vi "TEST_LvMarkdown.vi"() -> ()   [LabVIEW 2021, in "LvMarkdown.lvlib"]
uses:
  LvMarkdown.lvlib
  TEST_LvMarkdownStep.ctl
  LvMarkdown/LineBreak/LineBreak.lvclass
  C:/GitHub/LvMarkdown/src/LvMarkdown/IRenderable/IRenderable.lvclass
  LvMarkdown/Collection/Collection.lvclass
  LvMarkdown/Heading/Heading.lvclass
  C:/GitHub/LvMarkdown/src/LvMarkdown/Markdown.lvclass
  LvMarkdown/Heading/Heading.lvclass/Heading.ctl
  LvMarkdown/Paragraph/Paragraph.lvclass
  LvMarkdown/Line/Line.lvclass
  LvMarkdown/HorizontalRule/HorizontalRule.lvclass
  LvMarkdown/Code/Code.lvclass
  LvMarkdown/Bold/Bold.lvclass
  LvMarkdown/Italic/Italic.lvclass
  LvMarkdown/Blockquote/Blockquote.lvclass
  LvMarkdown/OrderedList/OrderedList.lvclass
  LvMarkdown/UnorderedList/UnorderedList.lvclass
  LvMarkdown/Image/Image.lvclass
  LvMarkdown/Image/Image.lvclass/Image.ctl
  LvMarkdown/Url/Url.lvclass
  LvMarkdown/Link/Link.lvclass
  LvMarkdown/Link/Link.lvclass/Link.ctl
  LvMarkdown/Table/Table.lvclass
  LvMarkdown/Alignment/AlignmentEnum.ctl
  LvMarkdown/Alignment/Alignment.lvclass
  LvMarkdown/Table/Table.lvclass/Table.ctl
  LvMarkdown/FencedCodeBlock/FencedCodeBlock.lvclass
  LvMarkdown/FencedCodeBlock/FencedCodeBlock.lvclass/FencedCodeBlock.ctl
  LvMarkdown/FootnoteReference/FootnoteReference.lvclass
  LvMarkdown/Footnote/Footnote.lvclass
  LvMarkdown/Footnote/Footnote.lvclass/Footnote.ctl
  b2edfd4d-23ef-4285-98b5-6188740e71bd.vi
  LvMarkdown/Heading/SetHeadingLevel.vi
  LvMarkdown/Image/SetTitle.vi
  LvMarkdown/Image/SetPath.vi
  LvMarkdown/Link/SetUrl.vi
  LvMarkdown/Table/SetTableRow.vi
  LvMarkdown/Table/SetAlignment.vi
  LvMarkdown/FencedCodeBlock/SetLanguage.vi
  LvMarkdown/Footnote/SetFootnoteReference.vi
  LvMarkdown/UnorderedList/SetUnorderedList.vi
  LvMarkdown/OrderedList/SetOrderedList.vi
  LvMarkdown/Table/SetHeader.vi
  <vilib>/ErrorRing/Error Ring.xnode
panel:
  out "String out":string
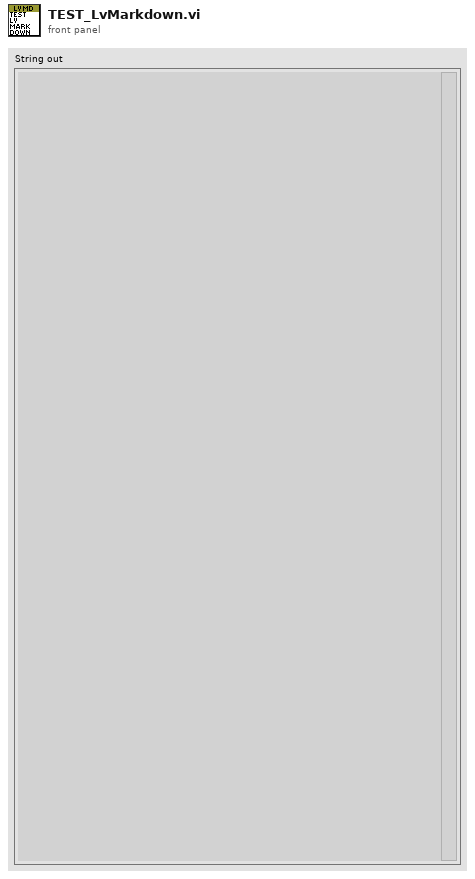
[diagram p1: front panel]
types:
  T1 = typedef "LvMarkdown.lvlib/TEST_LvMarkdownStep.ctl" = enum16{"Init", "Heading 1", "Paragraph 1", "Heading 2", "Paragraph 2", "Line", "Horizontal Rule", "Emphasis", "Blockquote", "List", "Image", "URL", "Link", "Table", "FencedCodeBlock", "Footnote", "Exit"}
  T2 = enum16{"Level 1", "Level 2", "Level 3", "Level 4", "Level 5", "Level 6"}
  T3 = typedef "LvMarkdown.lvlib/Alignment.lvclass/AlignmentEnum.ctl" = enum16{"Left", "Center", "Right"}
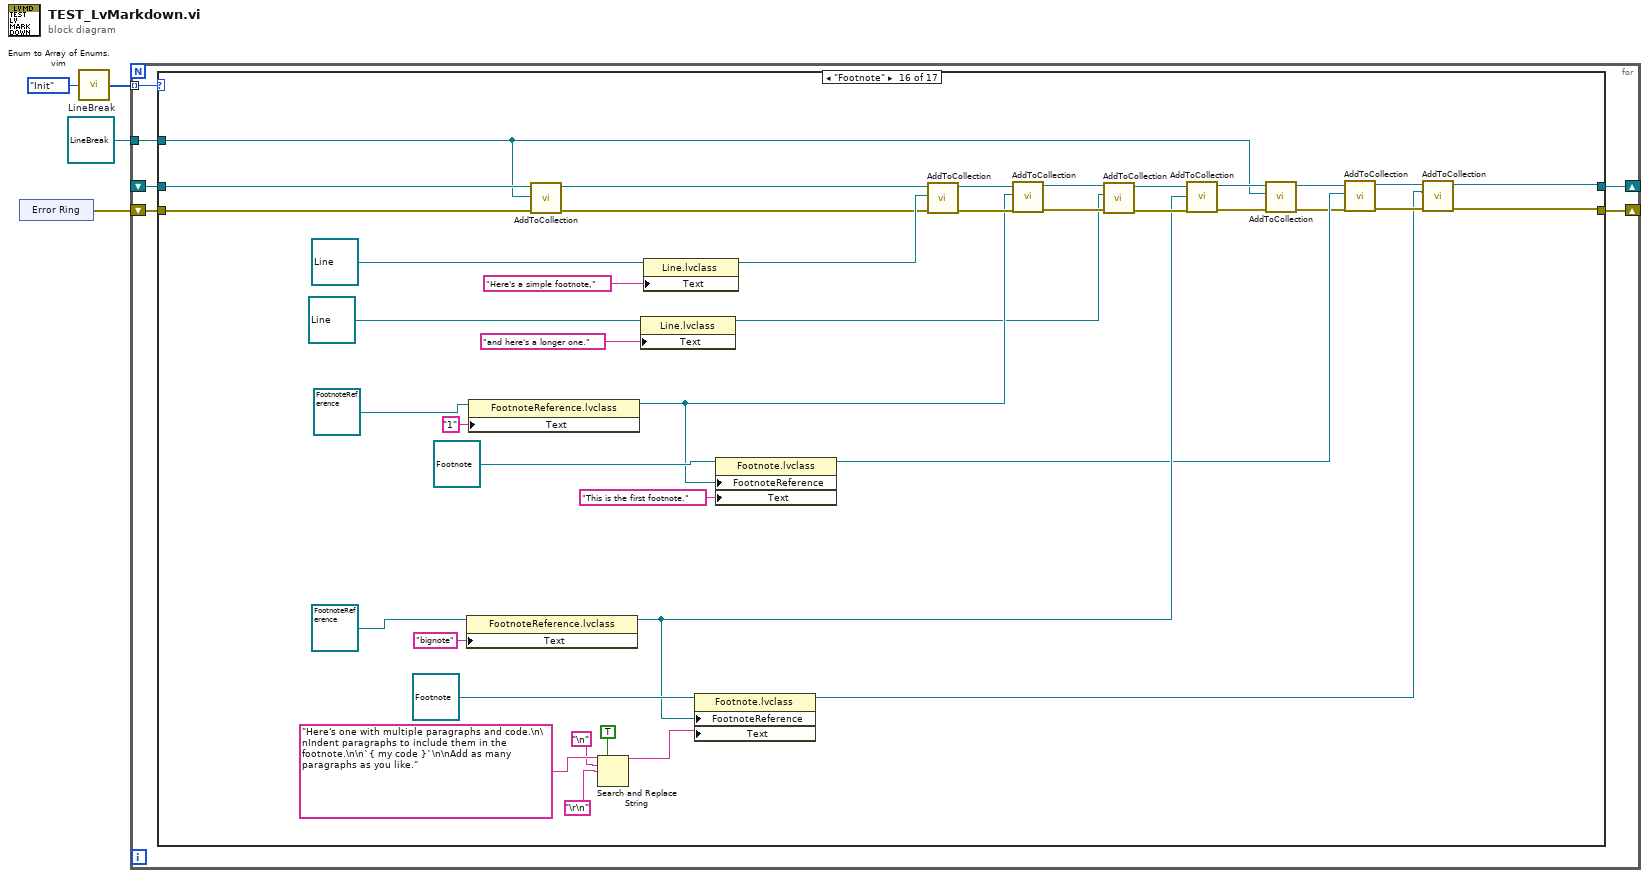
[diagram p0: block diagram]
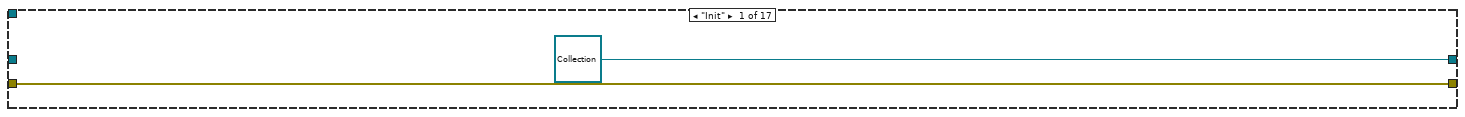
[diagram p2: hidden frame]
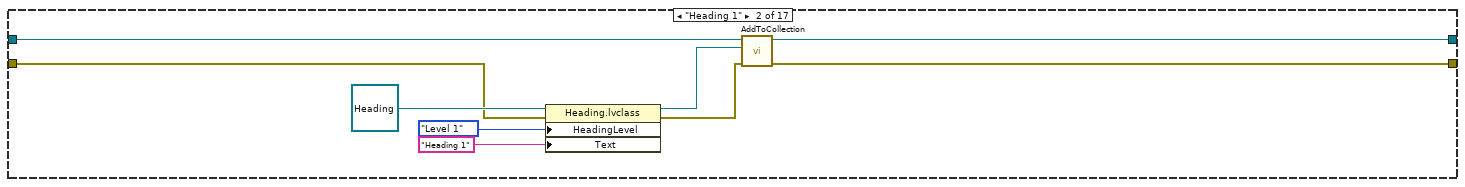
[diagram p3: hidden frame]
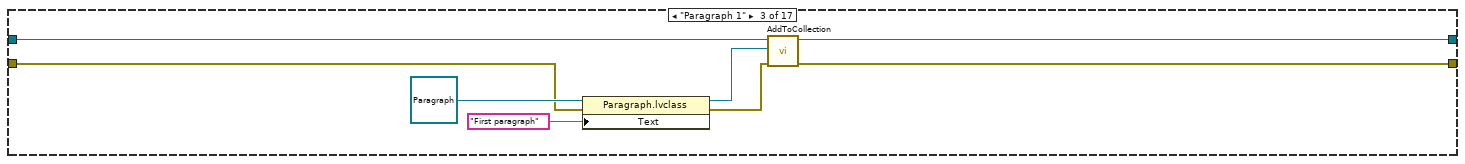
[diagram p4: hidden frame]
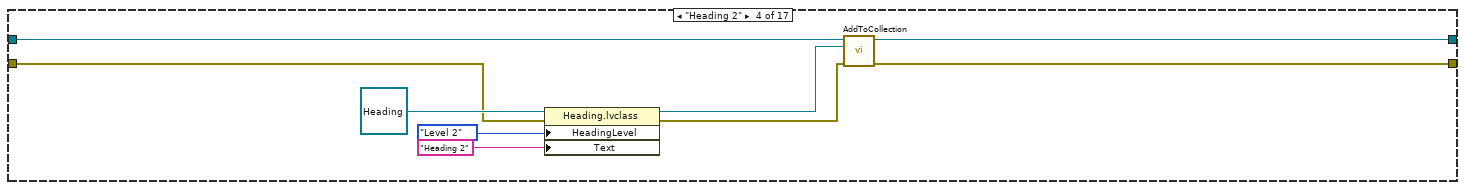
[diagram p5: hidden frame]
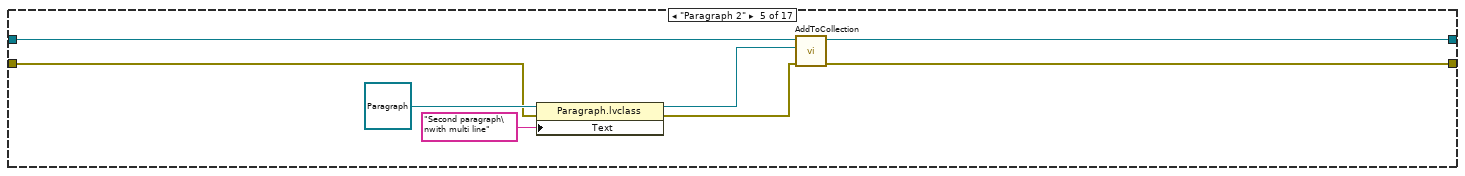
[diagram p6: hidden frame]
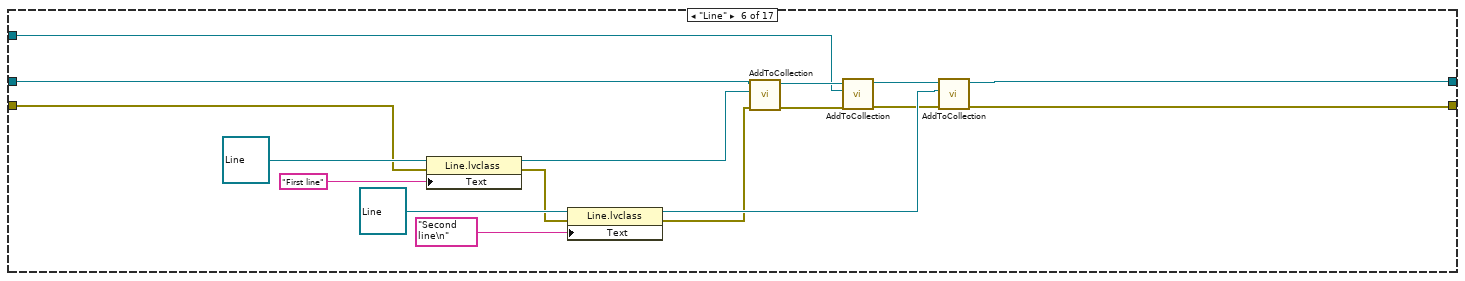
[diagram p7: hidden frame]
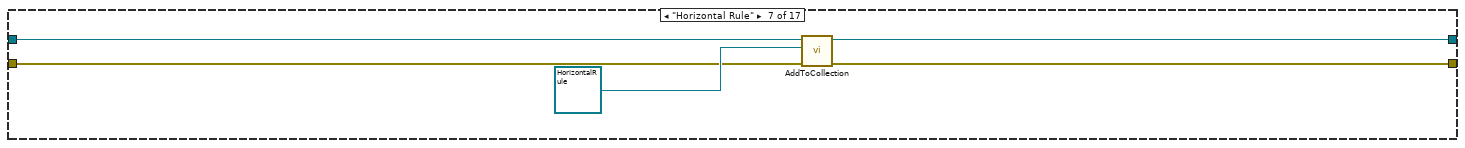
[diagram p8: hidden frame]
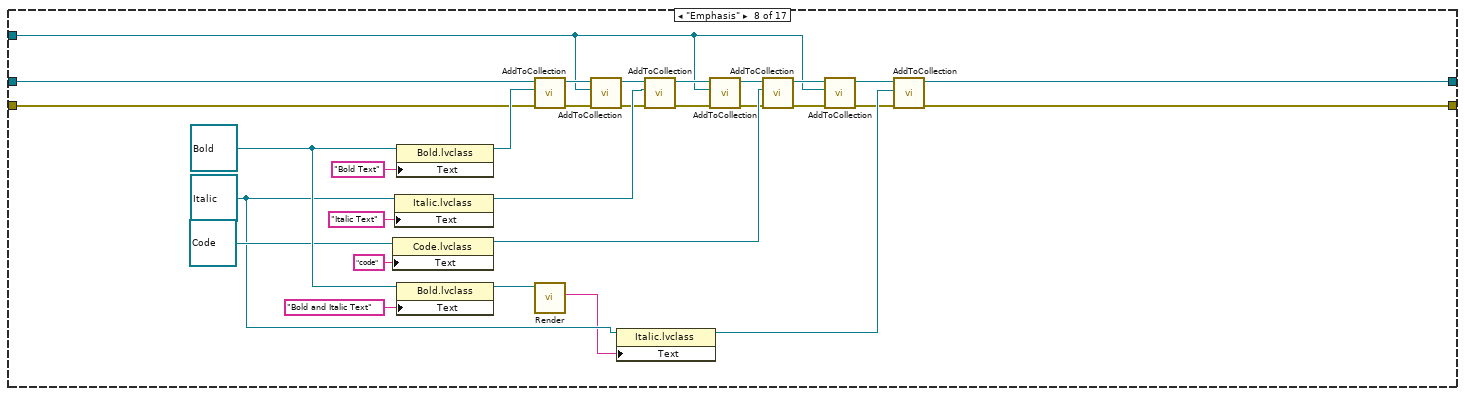
[diagram p9: hidden frame]
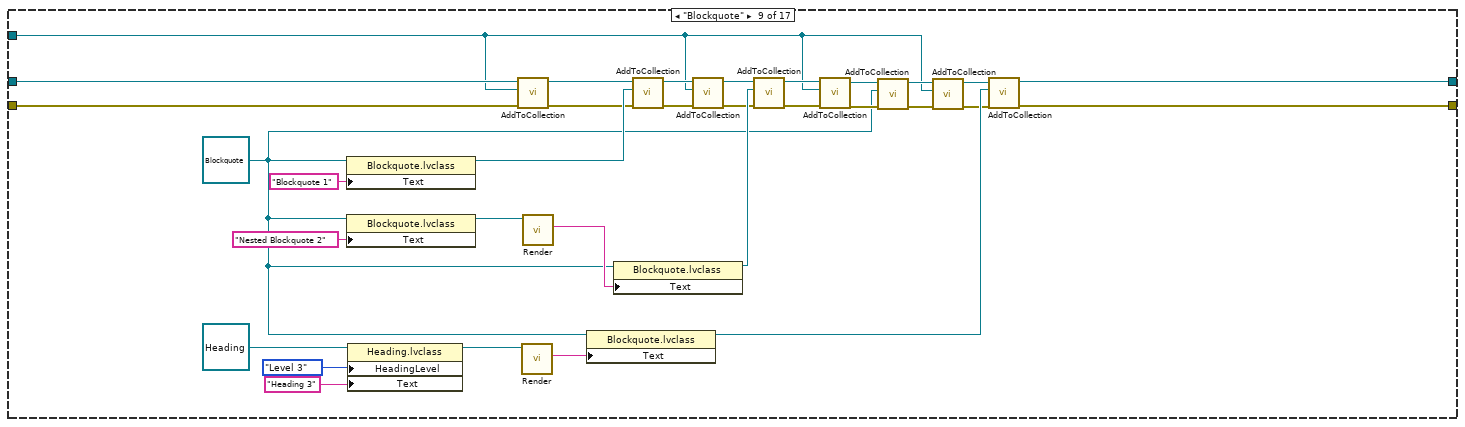
[diagram p10: hidden frame]
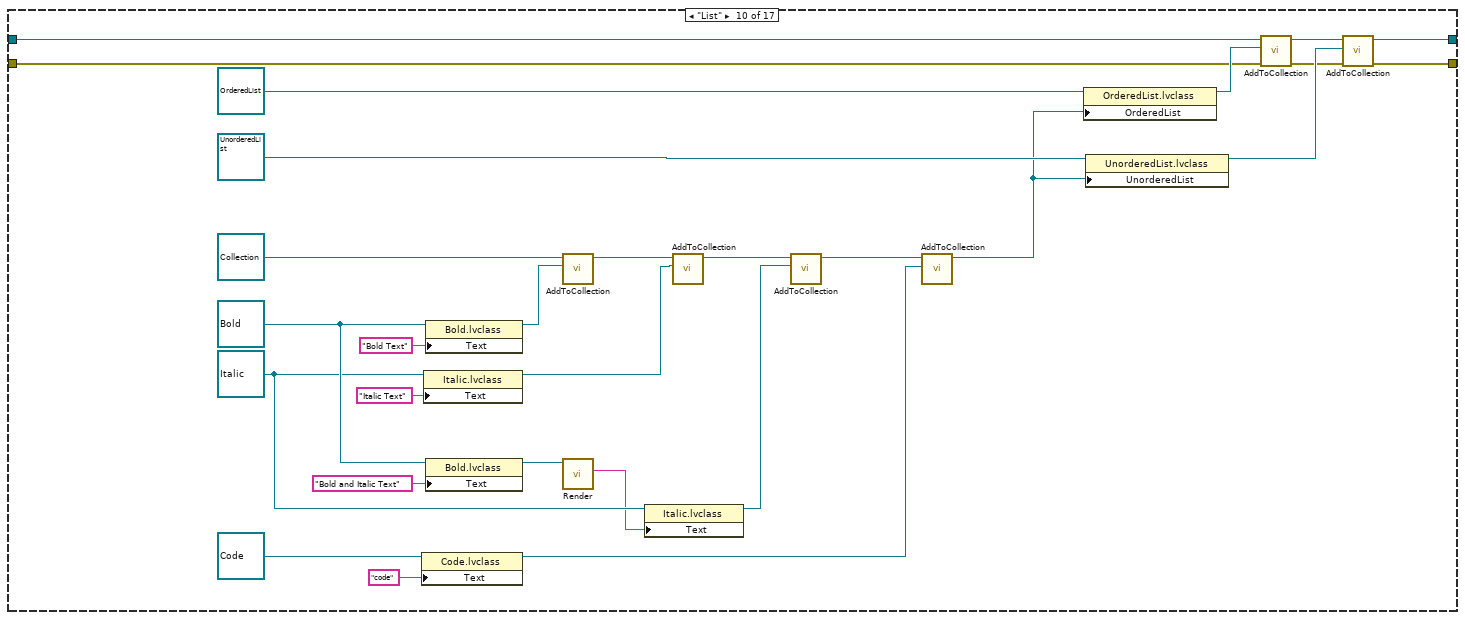
[diagram p11: hidden frame]
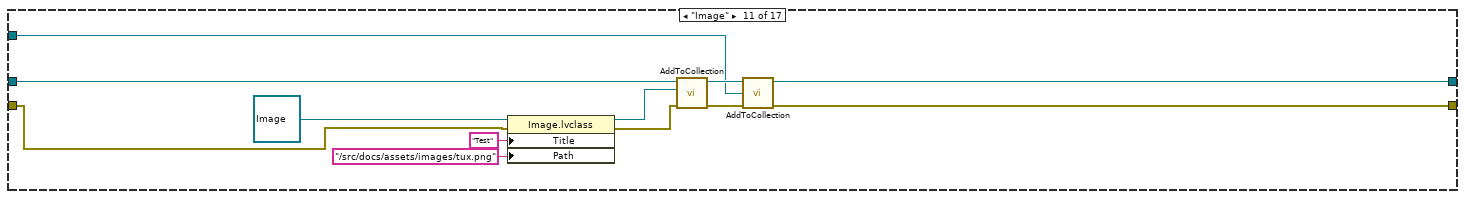
[diagram p12: hidden frame]
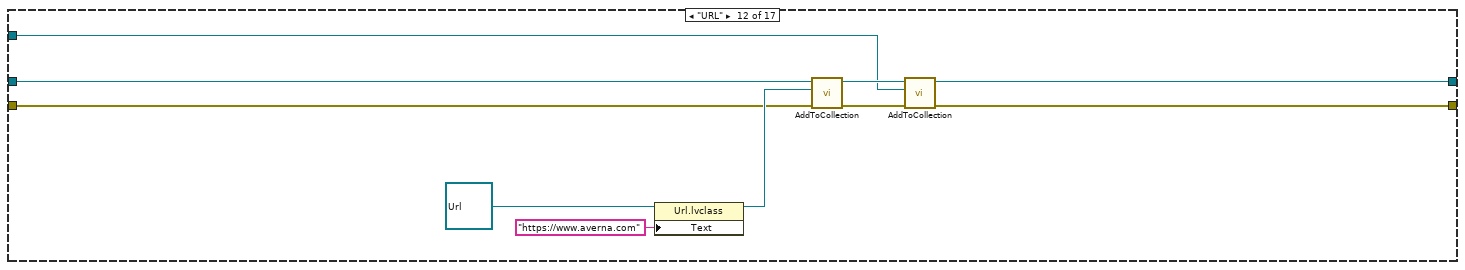
[diagram p13: hidden frame]
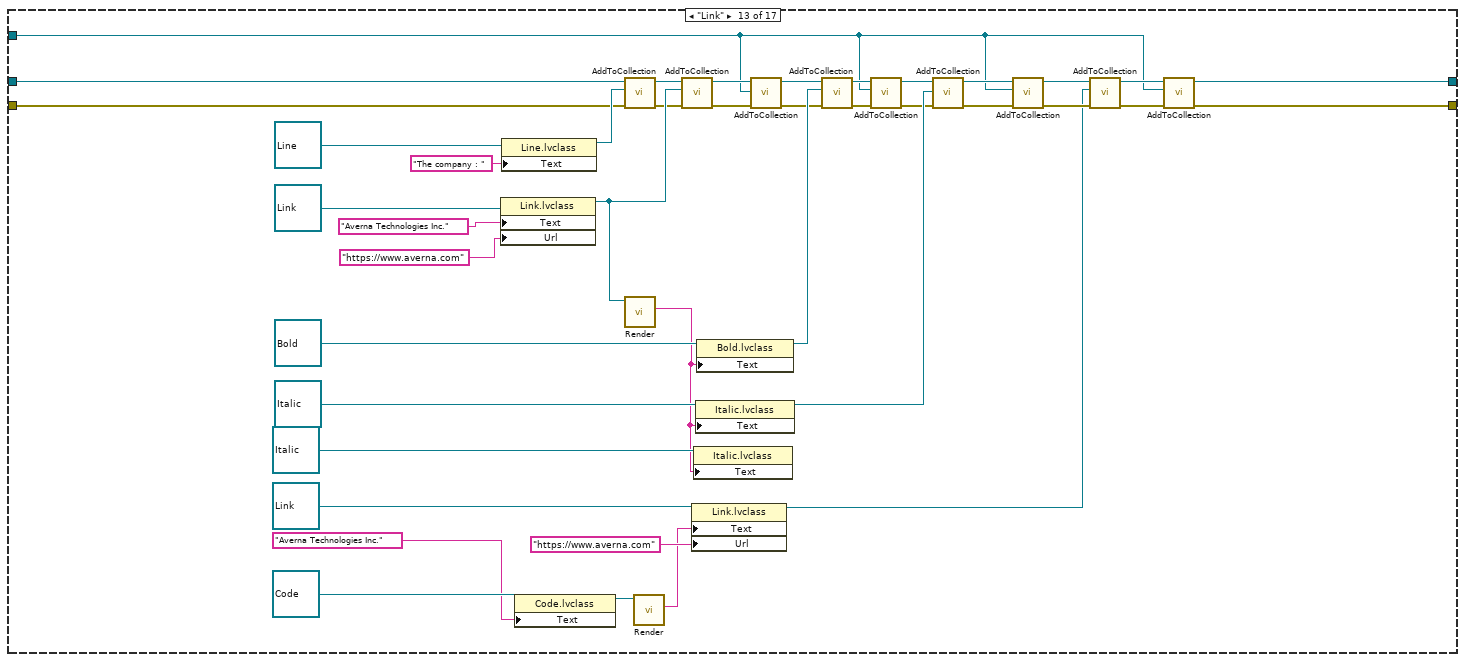
[diagram p14: hidden frame]
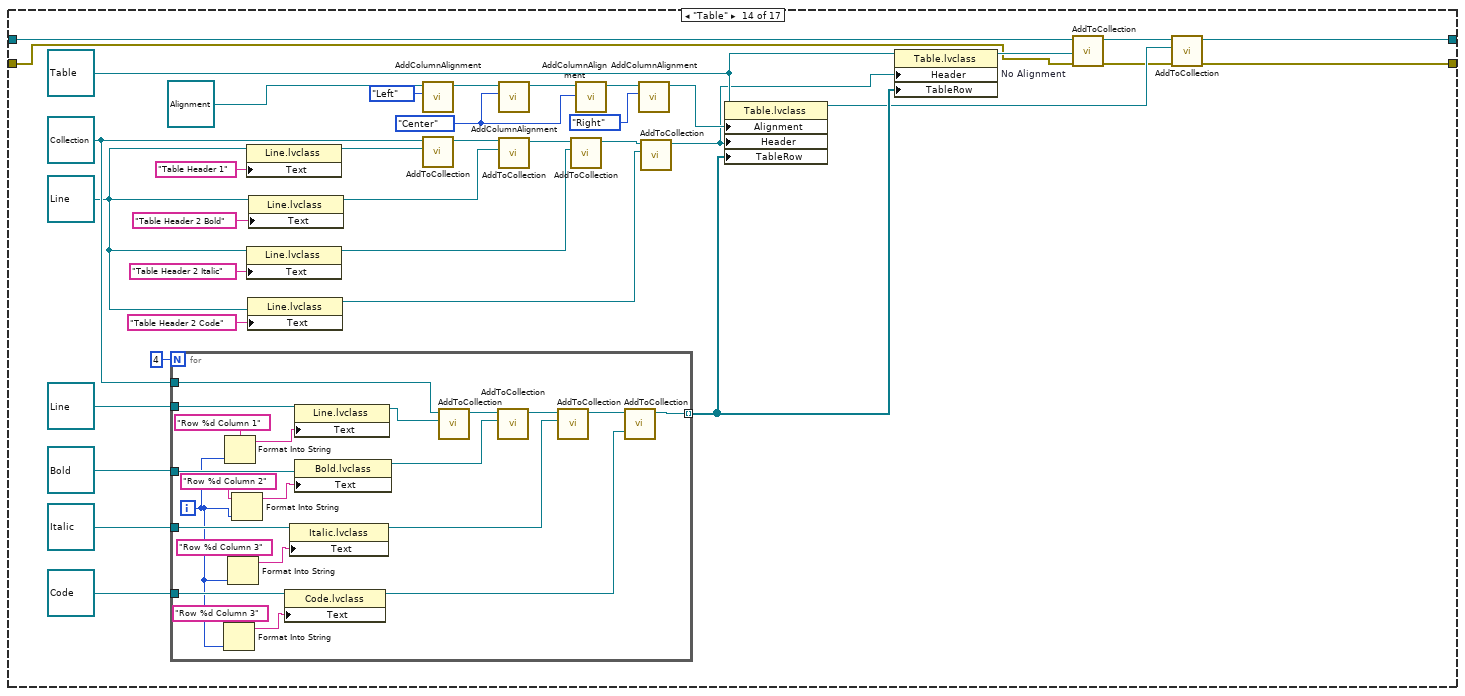
[diagram p15: hidden frame]
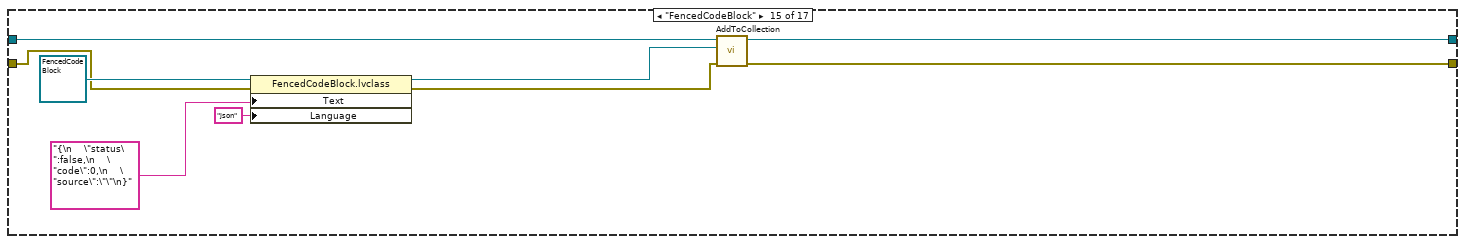
[diagram p16: hidden frame]
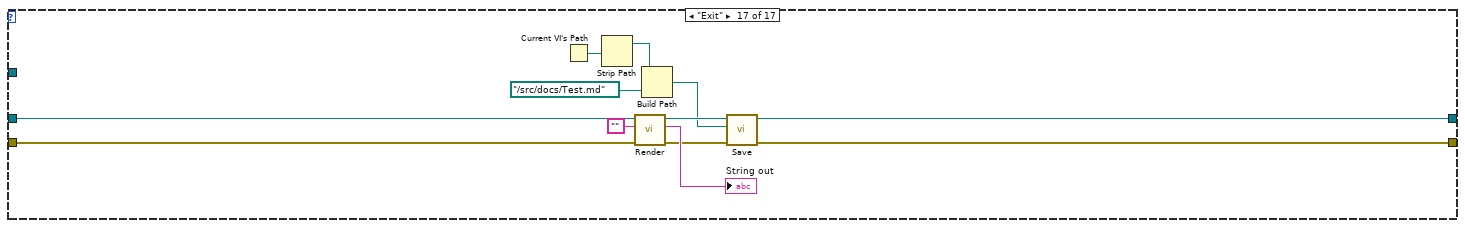
[diagram p17: hidden frame]
diagram:
  w2 = refnum<class "LineBreak.lvclass"> refnum  # LineBreak
  n1 = xnode "Error Ring"() -> ("error out"=w1:errorcluster)
  n2 = call "Enum to Array of Enums.vim"("enum"=TEST_LvMarkdownStep."Init") -> ("array of enums"=w4:T1[])
  n3 = for {
    tunnel: w4 -> [w10] mode=indexing
    shift-right: [w9] -> _
    shift-left: _ -> [w8]
    tunnel: w2 -> [w7]
    shift-right: [w5] -> _
    shift-left: w1 -> [w6]
    n4 = case shown="\"Footnote\"" w10 {
      tunnel: [refnum<class "Collection.lvclass"> refnum ("Markdown.lvlib:Collection.lvclass") w17 w26 w36 w44 w57 w68 w79 w115 w137 w164 w175 w184 w228 w285 w313 w334] -> w9
      tunnel: w8 -> [_ w18 w27 w35 w42 w59 w67 w89 w113 w156 w167 w178 w217 w225 w286 w300 w335]
      tunnel: w7 -> [_ _ _ _ _ w53 _ w77 w99 _ w163 w174 w181 _ _ w295 _]
      tunnel: w6 -> [w11 w14 w23 w31 w40 w47 w64 w69 w107 w131 w160 w171 w202 w222 w282 w330 w331]
      tunnel: [w11 w13 w22 w30 w39 w50 w65 w70 w108 w132 w159 w172 w182 w223 w281 w314 w332] -> w5
      frame "Init" {
      }
      frame "Heading 1" {
        n5 = property class="Heading.lvclass"(reference=refnum<class "Heading.lvclass"> refnum ("Markdown.lvlib:Heading.lvclass"), error in=w14, "HeadingLevel"=T2."Level 1", "Text"="Heading 1") -> (reference out=w16:refnum<class "Heading.lvclass">, error out=w15:errorcluster)
        n6 = call-dynamic "AddToCollection.vi"("error in (no error)"=w15, "IRenderable"=w16, "Collection in"=w18) -> ("error out"=w13:errorcluster, "Collection out"=w17:refnum<class "Collection.lvclass">)  [unwired: 7 in]
      }
      frame "Paragraph 1" {
        n7 = property class="Paragraph.lvclass"(reference=refnum<class "Paragraph.lvclass"> refnum ("Markdown.lvlib:Paragraph.lvclass"), error in=w23, "Text"="First paragraph") -> (reference out=w25:refnum<class "Paragraph.lvclass">, error out=w24:errorcluster)
        n8 = call-dynamic "AddToCollection.vi"("error in (no error)"=w24, "IRenderable"=w25, "Collection in"=w27) -> ("error out"=w22:errorcluster, "Collection out"=w26:refnum<class "Collection.lvclass">)  [unwired: 7 in]
      }
      frame "Heading 2" {
        n9 = property class="Heading.lvclass"(reference=refnum<class "Heading.lvclass"> refnum ("Markdown.lvlib:Heading.lvclass"), error in=w31, "HeadingLevel"=T2."Level 2" ("HeadingLevel 2"), "Text"="Heading 2") -> (reference out=w34:refnum<class "Heading.lvclass">, error out=w32:errorcluster)
        n10 = call-dynamic "AddToCollection.vi"("error in (no error)"=w32, "IRenderable"=w34, "Collection in"=w35) -> ("error out"=w30:errorcluster, "Collection out"=w36:refnum<class "Collection.lvclass">)  [unwired: 7 in]
      }
      frame "Paragraph 2" {
        n11 = property class="Paragraph.lvclass"(reference=refnum<class "Paragraph.lvclass"> refnum ("Markdown.lvlib:Paragraph.lvclass"), error in=w40, "Text"="Second paragraph\nwith multi line") -> (reference out=w43:refnum<class "Paragraph.lvclass">, error out=w41:errorcluster)
        n12 = call-dynamic "AddToCollection.vi"("error in (no error)"=w41, "IRenderable"=w43, "Collection in"=w42) -> ("error out"=w39:errorcluster, "Collection out"=w44:refnum<class "Collection.lvclass">)  [unwired: 7 in]
      }
      frame "Line" {
        n13 = property class="Line.lvclass"(reference=refnum<class "Line.lvclass"> refnum ("Markdown.lvlib:Line.lvclass"), error in=w47, "Text"="First line") -> (reference out=w56:refnum<class "Line.lvclass">, error out=w49:errorcluster)
        n14 = property class="Line.lvclass"(reference=refnum<class "Line.lvclass"> refnum ("Markdown.lvlib:Line.lvclass"), error in=w49, "Text"="Second line\n") -> (reference out=w55:refnum<class "Line.lvclass">, error out=w48:errorcluster)
        n15 = call-dynamic "AddToCollection.vi"("error in (no error)"=w48, "IRenderable"=w56, "Collection in"=w59) -> ("error out"=w52:errorcluster, "Collection out"=w58:refnum<class "Collection.lvclass">)  [unwired: 7 in]
        n16 = call-dynamic "AddToCollection.vi"("error in (no error)"=w52, "IRenderable"=w53, "Collection in"=w58) -> ("error out"=w51:errorcluster, "Collection out"=w54:refnum<class "Collection.lvclass">)  [unwired: 7 in]
        n17 = call-dynamic "AddToCollection.vi"("error in (no error)"=w51, "IRenderable"=w55, "Collection in"=w54) -> ("error out"=w50:errorcluster, "Collection out"=w57:refnum<class "Collection.lvclass">)  [unwired: 7 in]
      }
      frame "Horizontal Rule" {
        n18 = call-dynamic "AddToCollection.vi"("error in (no error)"=w64, "IRenderable"=refnum<class "HorizontalRule.lvclass"> refnum ("Markdown.lvlib:HorizontalRule.lvclass"), "Collection in"=w67) -> ("error out"=w65:errorcluster, "Collection out"=w68:refnum<class "Collection.lvclass">)  [unwired: 7 in]
      }
      frame "Emphasis" {
        w91 = refnum<class "Italic.lvclass"> refnum ("Markdown.lvlib:Italic.lvclass")
        w96 = refnum<class "Bold.lvclass"> refnum ("Markdown.lvlib:Bold.lvclass")
        n19 = property class="Code.lvclass"(reference=refnum<class "Code.lvclass"> refnum ("Markdown.lvlib:Code.lvclass"), "Text"="code") -> (reference out=w82:refnum<class "Code.lvclass">)  [unwired: 1 in, 1 out]
        n20 = property class="Italic.lvclass"(reference=w91, "Text"="Italic Text") -> (reference out=w85:refnum<class "Italic.lvclass">)  [unwired: 1 in, 1 out]
        n21 = property class="Bold.lvclass"(reference=w96, "Text"="Bold Text") -> (reference out=w87:refnum<class "Bold.lvclass">)  [unwired: 1 in, 1 out]
        n22 = property class="Bold.lvclass"(reference=w96, "Text"="Bold and Italic Text") -> (reference out=w95:refnum<class "Bold.lvclass">)  [unwired: 1 in, 1 out]
        n23 = call-dynamic "AddToCollection.vi"("error in (no error)"=w69, "IRenderable"=w87, "Collection in"=w89) -> ("error out"=w76:errorcluster, "Collection out"=w88:refnum<class "Collection.lvclass">)  [unwired: 7 in]
        n24 = call-dynamic "Render.vi"("Bold in"=w95) -> ("String out"=w90:string)  [unwired: 8 in, 2 out]
        n25 = call-dynamic "AddToCollection.vi"("error in (no error)"=w76, "IRenderable"=w77, "Collection in"=w88) -> ("error out"=w75:errorcluster, "Collection out"=w86:refnum<class "Collection.lvclass">)  [unwired: 7 in]
        n26 = property class="Italic.lvclass"(reference=w91, "Text"=w90) -> (reference out=w78:refnum<class "Italic.lvclass">)  [unwired: 1 in, 1 out]
        n27 = call-dynamic "AddToCollection.vi"("error in (no error)"=w75, "IRenderable"=w85, "Collection in"=w86) -> ("error out"=w74:errorcluster, "Collection out"=w84:refnum<class "Collection.lvclass">)  [unwired: 7 in]
        n28 = call-dynamic "AddToCollection.vi"("error in (no error)"=w74, "IRenderable"=w77, "Collection in"=w84) -> ("error out"=w73:errorcluster, "Collection out"=w83:refnum<class "Collection.lvclass">)  [unwired: 7 in]
        n29 = call-dynamic "AddToCollection.vi"("error in (no error)"=w73, "IRenderable"=w82, "Collection in"=w83) -> ("error out"=w72:errorcluster, "Collection out"=w80:refnum<class "Collection.lvclass">)  [unwired: 7 in]
        n30 = call-dynamic "AddToCollection.vi"("error in (no error)"=w72, "IRenderable"=w77, "Collection in"=w80) -> ("error out"=w71:errorcluster, "Collection out"=w81:refnum<class "Collection.lvclass">)  [unwired: 7 in]
        n31 = call-dynamic "AddToCollection.vi"("error in (no error)"=w71, "IRenderable"=w78, "Collection in"=w81) -> ("error out"=w70:errorcluster, "Collection out"=w79:refnum<class "Collection.lvclass">)  [unwired: 7 in]
      }
      frame "Blockquote" {
        w103 = refnum<class "Blockquote.lvclass"> refnum ("Markdown.lvlib:Blockquote.lvclass")
        n32 = property class="Blockquote.lvclass"(reference=w103, "Text"="Blockquote 1") -> (reference out=w125:refnum<class "Blockquote.lvclass">)  [unwired: 1 in, 1 out]
        n33 = property class="Blockquote.lvclass"(reference=w103, "Text"="Nested Blockquote 2") -> (reference out=w127:refnum<class "Blockquote.lvclass">)  [unwired: 1 in, 1 out]
        n34 = property class="Heading.lvclass"(reference=refnum<class "Heading.lvclass"> refnum ("Markdown.lvlib:Heading.lvclass"), "HeadingLevel"=T2."Level 3", "Text"="Heading 3") -> (reference out=w119:refnum<class "Heading.lvclass">)  [unwired: 1 in, 1 out]
        n35 = call-dynamic "AddToCollection.vi"("error in (no error)"=w107, "IRenderable"=w99, "Collection in"=w113) -> ("error out"=w112:errorcluster, "Collection out"=w114:refnum<class "Collection.lvclass">)  [unwired: 7 in]
        n36 = call-dynamic "Render.vi"("Heading in"=w119) -> ("String out"=w118:string)  [unwired: 8 in, 2 out]
        n37 = call-dynamic "Render.vi"("Blockquote in"=w127) -> ("String out"=w124:string)  [unwired: 8 in, 2 out]
        n38 = property class="Blockquote.lvclass"(reference=w103, "Text"=w118) -> (reference out=w116:refnum<class "Blockquote.lvclass">)  [unwired: 1 in, 1 out]
        n39 = property class="Blockquote.lvclass"(reference=w103, "Text"=w124) -> (reference out=w126:refnum<class "Blockquote.lvclass">)  [unwired: 1 in, 1 out]
        n40 = call-dynamic "AddToCollection.vi"("error in (no error)"=w112, "IRenderable"=w125, "Collection in"=w114) -> ("error out"=w111:errorcluster, "Collection out"=w123:refnum<class "Collection.lvclass">)  [unwired: 7 in]
        n41 = call-dynamic "AddToCollection.vi"("error in (no error)"=w111, "IRenderable"=w99, "Collection in"=w123) -> ("error out"=w110:errorcluster, "Collection out"=w128:refnum<class "Collection.lvclass">)  [unwired: 7 in]
        n42 = call-dynamic "AddToCollection.vi"("error in (no error)"=w110, "IRenderable"=w126, "Collection in"=w128) -> ("error out"=w109:errorcluster, "Collection out"=w117:refnum<class "Collection.lvclass">)  [unwired: 7 in]
        n43 = call-dynamic "AddToCollection.vi"("error in (no error)"=w109, "IRenderable"=w99, "Collection in"=w117) -> ("error out"=w106:errorcluster, "Collection out"=w105:refnum<class "Collection.lvclass">)  [unwired: 7 in]
        n44 = call-dynamic "AddToCollection.vi"("error in (no error)"=w106, "IRenderable"=w103, "Collection in"=w105) -> ("error out"=w104:errorcluster, "Collection out"=w101:refnum<class "Collection.lvclass">)  [unwired: 7 in]
        n45 = call-dynamic "AddToCollection.vi"("error in (no error)"=w104, "IRenderable"=w99, "Collection in"=w101) -> ("error out"=w102:errorcluster, "Collection out"=w100:refnum<class "Collection.lvclass">)  [unwired: 7 in]
        n46 = call-dynamic "AddToCollection.vi"("error in (no error)"=w102, "IRenderable"=w116, "Collection in"=w100) -> ("error out"=w108:errorcluster, "Collection out"=w115:refnum<class "Collection.lvclass">)  [unwired: 7 in]
      }
      frame "List" {
        w148 = refnum<class "Italic.lvclass"> refnum ("Markdown.lvlib:Italic.lvclass")
        w153 = refnum<class "Bold.lvclass"> refnum ("Markdown.lvlib:Bold.lvclass")
        n47 = property class="Code.lvclass"(reference=refnum<class "Code.lvclass"> refnum ("Markdown.lvlib:Code.lvclass"), "Text"="code") -> (reference out=w135:refnum<class "Code.lvclass">)  [unwired: 1 in, 1 out]
        n48 = property class="Italic.lvclass"(reference=w148, "Text"="Italic Text") -> (reference out=w145:refnum<class "Italic.lvclass">)  [unwired: 1 in, 1 out]
        n49 = property class="Bold.lvclass"(reference=w153, "Text"="Bold Text") -> (reference out=w146:refnum<class "Bold.lvclass">)  [unwired: 1 in, 1 out]
        n50 = property class="Bold.lvclass"(reference=w153, "Text"="Bold and Italic Text") -> (reference out=w152:refnum<class "Bold.lvclass">)  [unwired: 1 in, 1 out]
        n51 = call-dynamic "AddToCollection.vi"("IRenderable"=w146, "Collection in"=refnum<class "Collection.lvclass"> refnum) -> ("Collection out"=w141:refnum<class "Collection.lvclass">)  [unwired: 8 in, 1 out]
        n52 = call-dynamic "Render.vi"("Bold in"=w152) -> ("String out"=w147:string)  [unwired: 8 in, 2 out]
        n53 = property class="Italic.lvclass"(reference=w148, "Text"=w147) -> (reference out=w134:refnum<class "Italic.lvclass">)  [unwired: 1 in, 1 out]
        n54 = call-dynamic "AddToCollection.vi"("IRenderable"=w145, "Collection in"=w141) -> ("Collection out"=w144:refnum<class "Collection.lvclass">)  [unwired: 8 in, 1 out]
        n55 = call-dynamic "AddToCollection.vi"("IRenderable"=w134, "Collection in"=w144) -> ("Collection out"=w143:refnum<class "Collection.lvclass">)  [unwired: 8 in, 1 out]
        n56 = call-dynamic "AddToCollection.vi"("IRenderable"=w135, "Collection in"=w143) -> ("Collection out"=w140:refnum<class "Collection.lvclass">)  [unwired: 8 in, 1 out]
        n57 = property class="OrderedList.lvclass"(reference=refnum<class "OrderedList.lvclass"> refnum ("Markdown.lvlib:OrderedList.lvclass"), "OrderedList"=w140) -> (reference out=w139:refnum<class "OrderedList.lvclass">)  [unwired: 1 in, 1 out]
        n58 = property class="UnorderedList.lvclass"(reference=refnum<class "UnorderedList.lvclass"> refnum ("Markdown.lvlib:UnorderedList.lvclass"), "UnorderedList"=w140) -> (reference out=w136:refnum<class "UnorderedList.lvclass">)  [unwired: 1 in, 1 out]
        n59 = call-dynamic "AddToCollection.vi"("error in (no error)"=w131, "IRenderable"=w139, "Collection in"=w156) -> ("error out"=w133:errorcluster, "Collection out"=w138:refnum<class "Collection.lvclass">)  [unwired: 7 in]
        n60 = call-dynamic "AddToCollection.vi"("error in (no error)"=w133, "IRenderable"=w136, "Collection in"=w138) -> ("error out"=w132:errorcluster, "Collection out"=w137:refnum<class "Collection.lvclass">)  [unwired: 7 in]
      }
      frame "Image" {
        n61 = property class="Image.lvclass"(reference=refnum<class "Image.lvclass"> refnum ("Markdown.lvlib:Image.lvclass"), error in=w160, "Title"="Test", "Path"="/src/docs/assets/images/tux.png") -> (reference out=w168:refnum<class "Image.lvclass">, error out=w162:errorcluster)
        n62 = call-dynamic "AddToCollection.vi"("error in (no error)"=w162, "IRenderable"=w168, "Collection in"=w167) -> ("error out"=w161:errorcluster, "Collection out"=w166:refnum<class "Collection.lvclass">)  [unwired: 7 in]
        n63 = call-dynamic "AddToCollection.vi"("error in (no error)"=w161, "IRenderable"=w163, "Collection in"=w166) -> ("error out"=w159:errorcluster, "Collection out"=w164:refnum<class "Collection.lvclass">)  [unwired: 7 in]
      }
      frame "URL" {
        n64 = property class="Url.lvclass"(reference=refnum<class "Url.lvclass"> refnum ("Markdown.lvlib:Url.lvclass"), "Text"="https://www.averna.com") -> (reference out=w176:refnum<class "Url.lvclass">)  [unwired: 1 in, 1 out]
        n65 = call-dynamic "AddToCollection.vi"("error in (no error)"=w171, "IRenderable"=w176, "Collection in"=w178) -> ("error out"=w173:errorcluster, "Collection out"=w177:refnum<class "Collection.lvclass">)  [unwired: 7 in]
        n66 = call-dynamic "AddToCollection.vi"("error in (no error)"=w173, "IRenderable"=w174, "Collection in"=w177) -> ("error out"=w172:errorcluster, "Collection out"=w175:refnum<class "Collection.lvclass">)  [unwired: 7 in]
      }
      frame "Link" {
        n67 = property class="Link.lvclass"(reference=refnum<class "Link.lvclass"> refnum ("Markdown.lvlib:Link.lvclass"), "Text"="Averna Technologies Inc.", "Url"="https://www.averna.com" ("Text")) -> (reference out=w211:refnum<class "Link.lvclass">)  [unwired: 1 in, 1 out]
        n68 = property class="Line.lvclass"(reference=refnum<class "Line.lvclass"> refnum ("Markdown.lvlib:Line.lvclass"), "Text"="The company : ") -> (reference out=w216:refnum<class "Line.lvclass">)  [unwired: 1 in, 1 out]
        n69 = property class="Code.lvclass"(reference=refnum<class "Code.lvclass"> refnum ("Markdown.lvlib:Code.lvclass"), "Text"="Averna Technologies Inc.") -> (reference out=w188:refnum<class "Code.lvclass">)  [unwired: 1 in, 1 out]
        n70 = call-dynamic "AddToCollection.vi"("error in (no error)"=w202, "IRenderable"=w216, "Collection in"=w217) -> ("error out"=w201:errorcluster, "Collection out"=w215:refnum<class "Collection.lvclass">)  [unwired: 7 in]
        n71 = call-dynamic "Render.vi"("Link in"=w211) -> ("String out"=w193:string)  [unwired: 8 in, 2 out]
        n72 = call-dynamic "Render.vi"("Bold in"=w188) -> ("String out"=w187:string)  [unwired: 8 in, 2 out]
        n73 = call-dynamic "AddToCollection.vi"("error in (no error)"=w201, "IRenderable"=w211, "Collection in"=w215) -> ("error out"=w200:errorcluster, "Collection out"=w210:refnum<class "Collection.lvclass">)  [unwired: 7 in]
        n74 = property class="Link.lvclass"(reference=refnum<class "Link.lvclass"> refnum ("Markdown.lvlib:Link.lvclass"), "Text"=w187, "Url"="https://www.averna.com" ("Text")) -> (reference out=w186:refnum<class "Link.lvclass">)  [unwired: 1 in, 1 out]
        n75 = property class="Italic.lvclass"(reference=refnum<class "Italic.lvclass"> refnum ("Markdown.lvlib:Italic.lvclass"), "Text"=w193) -> ()  [unwired: 1 in, 2 out]
        n76 = property class="Italic.lvclass"(reference=refnum<class "Italic.lvclass"> refnum ("Markdown.lvlib:Italic.lvclass"), "Text"=w193) -> (reference out=w205:refnum<class "Italic.lvclass">)  [unwired: 1 in, 1 out]
        n77 = property class="Bold.lvclass"(reference=refnum<class "Bold.lvclass"> refnum ("Markdown.lvlib:Bold.lvclass"), "Text"=w193) -> (reference out=w206:refnum<class "Bold.lvclass">)  [unwired: 1 in, 1 out]
        n78 = call-dynamic "AddToCollection.vi"("error in (no error)"=w200, "IRenderable"=w181, "Collection in"=w210) -> ("error out"=w199:errorcluster, "Collection out"=w209:refnum<class "Collection.lvclass">)  [unwired: 7 in]
        n79 = call-dynamic "AddToCollection.vi"("error in (no error)"=w199, "IRenderable"=w206, "Collection in"=w209) -> ("error out"=w198:errorcluster, "Collection out"=w208:refnum<class "Collection.lvclass">)  [unwired: 7 in]
        n80 = call-dynamic "AddToCollection.vi"("error in (no error)"=w198, "IRenderable"=w181, "Collection in"=w208) -> ("error out"=w197:errorcluster, "Collection out"=w207:refnum<class "Collection.lvclass">)  [unwired: 7 in]
        n81 = call-dynamic "AddToCollection.vi"("error in (no error)"=w197, "IRenderable"=w205, "Collection in"=w207) -> ("error out"=w196:errorcluster, "Collection out"=w204:refnum<class "Collection.lvclass">)  [unwired: 7 in]
        n82 = call-dynamic "AddToCollection.vi"("error in (no error)"=w196, "IRenderable"=w181, "Collection in"=w204) -> ("error out"=w195:errorcluster, "Collection out"=w203:refnum<class "Collection.lvclass">)  [unwired: 7 in]
        n83 = call-dynamic "AddToCollection.vi"("error in (no error)"=w195, "IRenderable"=w186, "Collection in"=w203) -> ("error out"=w183:errorcluster, "Collection out"=w185:refnum<class "Collection.lvclass">)  [unwired: 7 in]
        n84 = call-dynamic "AddToCollection.vi"("error in (no error)"=w183, "IRenderable"=w181, "Collection in"=w185) -> ("error out"=w182:errorcluster, "Collection out"=w184:refnum<class "Collection.lvclass">)  [unwired: 7 in]
      }
      frame "Table" {
        w235 = AlignmentEnum."Center" ("Alignment")
        w253 = refnum<class "Collection.lvclass"> refnum ("Collection in")
        w245 = refnum<class "Line.lvclass"> refnum ("Markdown.lvlib:Line.lvclass")
        w232 = refnum<class "Table.lvclass"> refnum ("LvMarkdown.lvlib:Table.lvclass")
        n85 = for {
          N: 4 -> [_]
          tunnel: refnum<class "Bold.lvclass"> refnum ("Markdown.lvlib:Bold.lvclass") -> [w276]
          tunnel: w253 -> [w278]
          tunnel: [w263] -> w231 mode=indexing
          tunnel: refnum<class "Line.lvclass"> refnum ("Markdown.lvlib:Line.lvclass") -> [w271]
          tunnel: refnum<class "Italic.lvclass"> refnum ("Markdown.lvlib:Italic.lvclass") -> [w269]
          tunnel: refnum<class "Code.lvclass"> refnum ("Markdown.lvlib:Code.lvclass") -> [w266]
          i -> [w261]
          n86 = Format Into String(format string="Row %d Column 3" ("Text"), w261) -> (resulting string=w265:string)  [unwired: 2 in, 1 out]
          n87 = Format Into String(format string="Row %d Column 1" ("Text"), w261) -> (resulting string=w275:string)  [unwired: 2 in, 1 out]
          n88 = Format Into String(format string="Row %d Column 3" ("Text"), w261) -> (resulting string=w270:string)  [unwired: 2 in, 1 out]
          n89 = Format Into String(format string="Row %d Column 2" ("Text"), w261) -> (resulting string=w274:string)  [unwired: 2 in, 1 out]
          n90 = property class="Code.lvclass"(reference=w266, "Text"=w265) -> (reference out=w262:refnum<class "Code.lvclass">)  [unwired: 1 in, 1 out]
          n91 = property class="Italic.lvclass"(reference=w269, "Text"=w270) -> (reference out=w267:refnum<class "Italic.lvclass">)  [unwired: 1 in, 1 out]
          n92 = property class="Line.lvclass"(reference=w271, "Text"=w275) -> (reference out=w279:refnum<class "Line.lvclass">)  [unwired: 1 in, 1 out]
          n93 = property class="Bold.lvclass"(reference=w276, "Text"=w274) -> (reference out=w277:refnum<class "Bold.lvclass">)  [unwired: 1 in, 1 out]
          n94 = call-dynamic "AddToCollection.vi"("IRenderable"=w279, "Collection in"=w278) -> ("Collection out"=w280:refnum<class "Collection.lvclass">)  [unwired: 8 in, 1 out]
          n95 = call-dynamic "AddToCollection.vi"("IRenderable"=w277, "Collection in"=w280) -> ("Collection out"=w268:refnum<class "Collection.lvclass">)  [unwired: 8 in, 1 out]
          n96 = call-dynamic "AddToCollection.vi"("IRenderable"=w267, "Collection in"=w268) -> ("Collection out"=w264:refnum<class "Collection.lvclass">)  [unwired: 8 in, 1 out]
          n97 = call-dynamic "AddToCollection.vi"("IRenderable"=w262, "Collection in"=w264) -> ("Collection out"=w263:refnum<class "Collection.lvclass">)  [unwired: 8 in, 1 out]
        }
        n98 = property class="Line.lvclass"(reference=w245, "Text"="Table Header 1") -> (reference out=w255:refnum<class "Line.lvclass">)  [unwired: 1 in, 1 out]
        n99 = property class="Line.lvclass"(reference=w245, "Text"="Table Header 2 Italic") -> (reference out=w242:refnum<class "Line.lvclass">)  [unwired: 1 in, 1 out]
        n100 = property class="Line.lvclass"(reference=w245, "Text"="Table Header 2 Code") -> (reference out=w241:refnum<class "Line.lvclass">)  [unwired: 1 in, 1 out]
        n101 = property class="Line.lvclass"(reference=w245, "Text"="Table Header 2 Bold") -> (reference out=w256:refnum<class "Line.lvclass">)  [unwired: 1 in, 1 out]
        n102 = call "AddColumnAlignment.vi"("Alignment"=AlignmentEnum."Left", "Alignment in"=refnum<class "Alignment.lvclass"> refnum ("LvMarkdown.lvlib:Alignment.lvclass")) -> ("Alignment out"=w240:refnum<class "Alignment.lvclass">)  [unwired: 8 in, 1 out]
        n103 = call-dynamic "AddToCollection.vi"("IRenderable"=w255, "Collection in"=w253) -> ("Collection out"=w254:refnum<class "Collection.lvclass">)  [unwired: 8 in, 1 out]
        n104 = call "AddColumnAlignment.vi"("Alignment"=w235, "Alignment in"=w240) -> ("Alignment out"=w239:refnum<class "Alignment.lvclass">)  [unwired: 8 in, 1 out]
        n105 = call-dynamic "AddToCollection.vi"("IRenderable"=w256, "Collection in"=w254) -> ("Collection out"=w243:refnum<class "Collection.lvclass">)  [unwired: 8 in, 1 out]
        n106 = call-dynamic "AddToCollection.vi"("IRenderable"=w242, "Collection in"=w243) -> ("Collection out"=w244:refnum<class "Collection.lvclass">)  [unwired: 8 in, 1 out]
        n107 = call "AddColumnAlignment.vi"("Alignment"=w235, "Alignment in"=w239) -> ("Alignment out"=w238:refnum<class "Alignment.lvclass">)  [unwired: 8 in, 1 out]
        n108 = call "AddColumnAlignment.vi"("Alignment"=AlignmentEnum."Right", "Alignment in"=w238) -> ("Alignment out"=w237:refnum<class "Alignment.lvclass">)  [unwired: 8 in, 1 out]
        n109 = call-dynamic "AddToCollection.vi"("IRenderable"=w241, "Collection in"=w244) -> ("Collection out"=w230:refnum<class "Collection.lvclass">)  [unwired: 8 in, 1 out]
        n110 = property class="Table.lvclass"(reference=w232, "Alignment"=w237, "Header"=w230, "TableRow"=w231) -> (reference out=w227:refnum<class "Table.lvclass">)  [unwired: 1 in, 1 out]
        n111 = property on="No Alignment" class="Table.lvclass"(reference=w232, "Header"=w230, "TableRow"=w231) -> (reference out=w226:refnum<class "Table.lvclass">)  [unwired: 1 in, 1 out]
        n112 = call-dynamic "AddToCollection.vi"("error in (no error)"=w222, "IRenderable"=w226, "Collection in"=w225) -> ("error out"=w224:errorcluster, "Collection out"=w229:refnum<class "Collection.lvclass">)  [unwired: 7 in]
        n113 = call-dynamic "AddToCollection.vi"("error in (no error)"=w224, "IRenderable"=w227, "Collection in"=w229) -> ("error out"=w223:errorcluster, "Collection out"=w228:refnum<class "Collection.lvclass">)  [unwired: 7 in]
      }
      frame "FencedCodeBlock" {
        n114 = property class="FencedCodeBlock.lvclass"(reference=refnum<class "FencedCodeBlock.lvclass"> refnum ("LvMarkdown.lvlib:FencedCodeBlock.lvclass"), error in=w282, "Text"="{\n    \"status\":false,\n    \"code\":0,\n    \"source\":\"\"\n}", "Language"="json") -> (reference out=w284:refnum<class "FencedCodeBlock.lvclass">, error out=w283:errorcluster)
        n115 = call-dynamic "AddToCollection.vi"("error in (no error)"=w283, "IRenderable"=w284, "Collection in"=w286) -> ("error out"=w281:errorcluster, "Collection out"=w285:refnum<class "Collection.lvclass">)  [unwired: 7 in]
      }
      frame "Footnote" {
        n116 = property class="FootnoteReference.lvclass"(reference=refnum<class "FootnoteReference.lvclass"> refnum ("LvMarkdown.lvlib:FootnoteReference.lvclass"), "Text"="bignote") -> (reference out=w305:refnum<class "FootnoteReference.lvclass">)  [unwired: 1 in, 1 out]
        n117 = property class="FootnoteReference.lvclass"(reference=refnum<class "FootnoteReference.lvclass"> refnum ("LvMarkdown.lvlib:FootnoteReference.lvclass"), "Text"="1") -> (reference out=w312:refnum<class "FootnoteReference.lvclass">)  [unwired: 1 in, 1 out]
        n118 = call-dynamic "AddToCollection.vi"("error in (no error)"=w330, "IRenderable"=w295, "Collection in"=w300) -> ("error out"=w301:errorcluster, "Collection out"=w299:refnum<class "Collection.lvclass">)  [unwired: 7 in]
        n119 = Search and Replace String(replace all?=TRUE ("replace all? (F)"), input string="Here's one with multiple paragraphs and code.\n\nIndent paragraphs to include them in the footnote.\n\n`{ my code }`\n\nAdd as many paragraphs as you like.", search string="\n", replace string="\r\n") -> (result string=w293:string)  [unwired: 4 in, 3 out]
        n120 = property class="Line.lvclass"(reference=refnum<class "Line.lvclass"> refnum ("LvMarkdown.lvlib:Line.lvclass"), "Text"="and here's a longer one.") -> (reference out=w309:refnum<class "Line.lvclass">)  [unwired: 1 in, 1 out]
        n121 = property class="Line.lvclass"(reference=refnum<class "Line.lvclass"> refnum ("LvMarkdown.lvlib:Line.lvclass"), "Text"="Here's a simple footnote,") -> (reference out=w324:refnum<class "Line.lvclass">)  [unwired: 1 in, 1 out]
        n122 = property class="Footnote.lvclass"(reference=refnum<class "Footnote.lvclass"> refnum ("LvMarkdown.lvlib:Footnote.lvclass"), "FootnoteReference"=w305, "Text"=w293) -> (reference out=w303:refnum<class "Footnote.lvclass">)  [unwired: 1 in, 1 out]
        n123 = property class="Footnote.lvclass"(reference=refnum<class "Footnote.lvclass"> refnum ("LvMarkdown.lvlib:Footnote.lvclass"), "FootnoteReference"=w312, "Text"="This is the first footnote.") -> (reference out=w304:refnum<class "Footnote.lvclass">)  [unwired: 1 in, 1 out]
        n124 = call-dynamic "AddToCollection.vi"("error in (no error)"=w301, "IRenderable"=w324, "Collection in"=w299) -> ("error out"=w322:errorcluster, "Collection out"=w323:refnum<class "Collection.lvclass">)  [unwired: 7 in]
        n125 = call-dynamic "AddToCollection.vi"("error in (no error)"=w322, "IRenderable"=w312, "Collection in"=w323) -> ("error out"=w320:errorcluster, "Collection out"=w321:refnum<class "Collection.lvclass">)  [unwired: 7 in]
        n126 = call-dynamic "AddToCollection.vi"("error in (no error)"=w320, "IRenderable"=w309, "Collection in"=w321) -> ("error out"=w318:errorcluster, "Collection out"=w319:refnum<class "Collection.lvclass">)  [unwired: 7 in]
        n127 = call-dynamic "AddToCollection.vi"("error in (no error)"=w318, "IRenderable"=w305, "Collection in"=w319) -> ("error out"=w317:errorcluster, "Collection out"=w297:refnum<class "Collection.lvclass">)  [unwired: 7 in]
        n128 = call-dynamic "AddToCollection.vi"("error in (no error)"=w317, "IRenderable"=w295, "Collection in"=w297) -> ("error out"=w298:errorcluster, "Collection out"=w296:refnum<class "Collection.lvclass">)  [unwired: 7 in]
        n129 = call-dynamic "AddToCollection.vi"("error in (no error)"=w298, "IRenderable"=w304, "Collection in"=w296) -> ("error out"=w315:errorcluster, "Collection out"=w316:refnum<class "Collection.lvclass">)  [unwired: 7 in]
        n130 = call-dynamic "AddToCollection.vi"("error in (no error)"=w315, "IRenderable"=w303, "Collection in"=w316) -> ("error out"=w314:errorcluster, "Collection out"=w313:refnum<class "Collection.lvclass">)  [unwired: 7 in]
      }
      frame "Exit" {
        n131 = Current VI's Path() -> (path=w339:path)
        n132 = Strip Path(path=w339) -> (stripped path=w338:path)  [unwired: 1 out]
        n133 = call-dynamic "Render.vi"("error in (no error)"=w331, "String in"="", "Collection in"=w335) -> ("error out"=w333:errorcluster, "String out"=→"String out":string, "Collection out"=w340:refnum<class "Collection.lvclass">)  [unwired: 6 in]
        n134 = Build Path(base path=w338, name or relative path=path "../src/docs/Test.md") -> (appended path=w337:path)
        n135 = call "Save.vi"("error in (no error)"=w333, "Path"=w337, "Collection in"=w340) -> ("error out"=w332:errorcluster, "Collection out"=w334:refnum<class "Collection.lvclass">)  [unwired: 7 in]
      }
    }
  }
